vi "Sequence.SeperateMainSections.vi"(8 "error in (no error)":errorcluster, 10 "UI.Sequence#ofColumns":i32, 11 "MulticolumnListbox in":refnum<vi>) -> (0 "error out":errorcluster, 1 "Conditions":string[][](array[string]), 2 "Duration":string[](array[string]), 3 "Steps":string[][](array[string]))   [LabVIEW 2013, in "Simple Sequence Editor.lvlib"]
uses:
  Simple Sequence Editor.lvlib
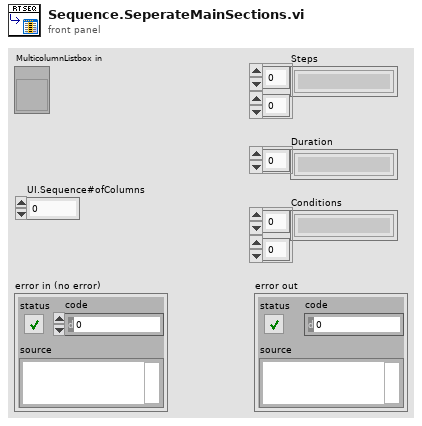
[diagram p1: front panel]
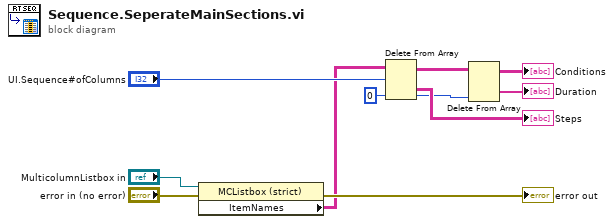
[diagram p0: block diagram]
diagram:
  w1 = 0 ("disabled index (col)")
  n1 = property class="MCListbox (strict)"(reference="MulticolumnListbox in", error in="error in (no error)") -> (error out=→"error out":errorcluster, "ItemNames"=w3:string[][])  [unwired: 1 out]
  n2 = Delete From Array(array=w3, length="UI.Sequence#ofColumns", index (col)=w1) -> (deleted portion=→"Steps":string[][], array with subset deleted=w2:string[][])  [unwired: 1 in]
  n3 = Delete From Array(array=w2, index (col)=w1) -> (deleted portion=→"Duration":string[], array with subset deleted=→"Conditions":string[][])  [unwired: 2 in]
